vi "CAN Parameters FG.vi"(7 "Action":T1, 8 "error in (no error)":errorcluster, 10 "Diagnostics Basic Configuraiton":T2={"Database File"=path "", "CAN Interface"=enum."CAN0", "Baud Rate"=0, "Diagnostic Protocol"=enum."GMLAN", "Transport Protocol"=enum."ISO TP - Normal Mode", "Transmit ID"=0, "Receive ID"=0, "Transmit Extension"=0, "Receive Extension"=0, "Receive UUDT ID"=0, "Enable Stream"=TRUE, "VW TP Channel ID"=0, "Security"={"Source DLL Path"=path "", "Security Level"=1, "Target DLL Path"=path ""}, "Fill Frame"=TRUE, "Fill Byte"=255, "Termination"=FALSE} {"Fill Byte" format="%.0x"; "VW TP Channel ID" format="%.0x"; "Receive UUDT ID" format="%.0x"; "Receive Extension" format="%.0x"; "Transmit Extension" format="%.0x"; "Receive ID" format="%.0x"; "Transmit ID" format="%.0x"}, 11 "Device Item Ref in":T7 format="%.0x") -> (0 "error out":errorcluster, 2 "Diagnostics Basic Configuraiton":T2={"Database File"=path "", "CAN Interface"=enum."CAN0", "Baud Rate"=0, "Diagnostic Protocol"=enum."GMLAN", "Transport Protocol"=enum."ISO TP - Normal Mode", "Transmit ID"=0, "Receive ID"=0, "Transmit Extension"=0, "Receive Extension"=0, "Receive UUDT ID"=0, "Enable Stream"=TRUE, "VW TP Channel ID"=0, "Security"={"Source DLL Path"=path "", "Security Level"=1, "Target DLL Path"=path ""}, "Fill Frame"=FALSE, "Fill Byte"=255, "Termination"=FALSE} {"Fill Byte" format="%.0x"; "VW TP Channel ID" format="%.0x"; "Receive UUDT ID" format="%.0x"; "Receive Extension" format="%.0x"; "Transmit Extension" format="%.0x"; "Receive ID" format="%.0x"; "Transmit ID" format="%.0x"}, 3 "Device Item Ref out":T7=18446744073709551615 format="%.0x")   [LabVIEW 2015, in "Diagnostics Addon System Explorer.lvlib"]
uses:
  System Explorer/Diagnostics Addon System Explorer.lvlib
  <vilib>/NI Veristand/Custom Device API/Custom Device Item Ref.ctl
  CAN Configuration.ctl
  CAN Interface.ctl
  Diagnostic Protocols.ctl
  Transport Protocols.ctl
  Security.ctl
  FG Action.ctl
  <vilib>/NI Veristand/Custom Device API/Set Item Property (Boolean).vi
  <vilib>/NI Veristand/Custom Device API/Set Item Property (U32).vi
  <vilib>/NI Veristand/Custom Device API/NI VeriStand - Remove Item Property.vi
  <vilib>/NI Veristand/Custom Device API/Set Item Property (Dependent File).vi
  <vilib>/Utility/MD5Checksum.llb/MD5Checksum File.vi
  GUID Lookup.vi
  <vilib>/NI Veristand/Custom Device API/Set Item Property (Path).vi
  <vilib>/NI Veristand/Custom Device API/Get Item Property (Boolean).vi
  <vilib>/NI Veristand/Custom Device API/Get Item Property (U32).vi
  <vilib>/NI Veristand/Custom Device API/Get Item Property (Path).vi
  Diagnostics Addon Shared.lvlib
  <vilib>/NI Veristand/Custom Device API/Custom Device API.lvlib
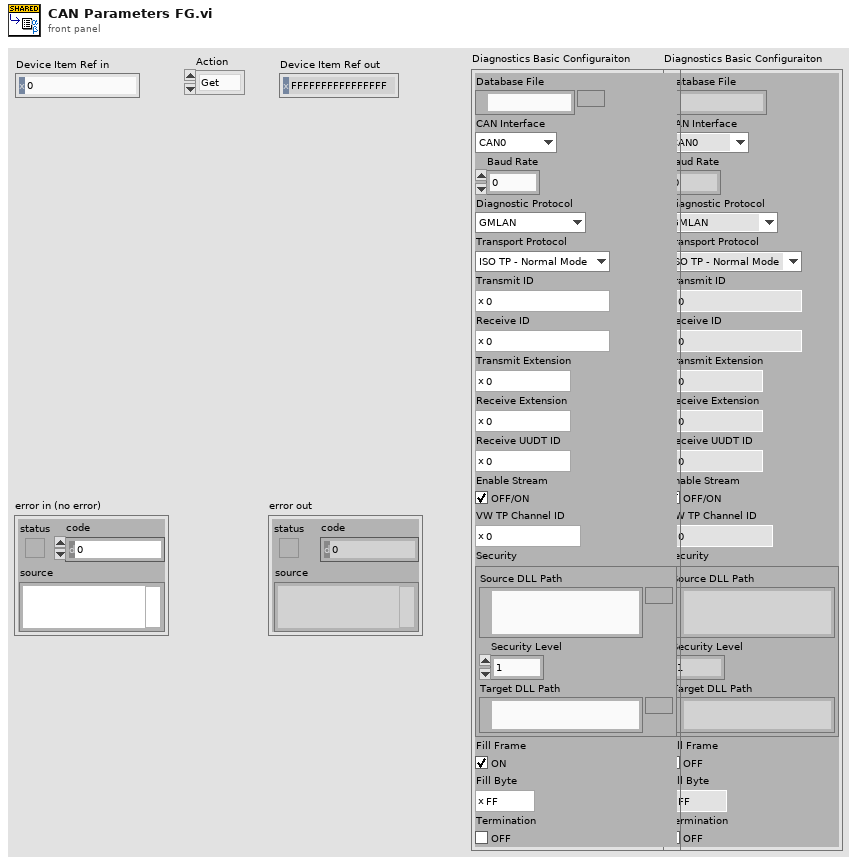
[diagram p1: front panel]
types:
  T1 = typedef "Diagnostics Addon System Explorer.lvlib/FG Action.ctl" = enum16{"Get", "Set"}
  T2 = typedef "Diagnostics Addon Shared.lvlib/CAN Configuration.ctl" = cluster{"Database File":path, "CAN Interface":T3, "Baud Rate":u32, "Diagnostic Protocol":T4, "Transport Protocol":T5, "Transmit ID":u32, "Receive ID":u32, "Transmit Extension":u8, "Receive Extension":u8, "Receive UUDT ID":u32, "Enable Stream":bool, "VW TP Channel ID":u32, "Security":T6, "Fill Frame":bool, "Fill Byte":u8, "Termination":bool}
  T3 = typedef "Diagnostics Addon Shared.lvlib/CAN Interface.ctl" = enum16{"CAN0", "CAN1", "CAN2", "CAN3", "CAN4", "CAN5", "CAN6", "CAN7", "CAN8", "CAN9", "CAN10", "CAN11", "CAN12", "CAN13", "CAN14", "CAN15", "CAN16", "CAN17", "CAN18", "CAN19", "CAN20", "CAN21", "CAN22", "CAN23", "CAN24", "CAN25", "CAN26", "CAN27", "CAN28", "CAN29", "CAN30", "CAN31", "CAN32", "CAN33", "CAN34", "CAN35", "CAN36", "CAN37", "CAN38", "CAN39", "CAN40", "CAN41", "CAN42", "CAN43", "CAN44", "CAN45", "CAN46", "CAN47", "CAN48", "CAN49", "CAN50", "CAN51", "CAN52", "CAN53", "CAN54", "CAN55", "CAN56", "CAN57", "CAN58", "CAN59", "CAN60", "CAN61", "CAN62", "CAN63", "CAN 256 (Virtual)", "CAN 257 (Virtual)"}
  T4 = typedef "Diagnostics Addon Shared.lvlib/Diagnostic Protocols.ctl" = enum16{"GMLAN", "KWP-2000", "UDS"}
  T5 = typedef "Diagnostics Addon Shared.lvlib/Transport Protocols.ctl" = enum16{"ISO TP - Normal Mode", "ISO TP - Mixed Mode", "VW TP 2.0", "Diagnostics on IP"}
  T6 = typedef "Diagnostics Addon Shared.lvlib/Security.ctl" = cluster{"Source DLL Path":path, "Security Level":u8, "Target DLL Path":path}
  T7 = typedef "Custom Device API.lvlib/Custom Device Item Ref.ctl" = u64
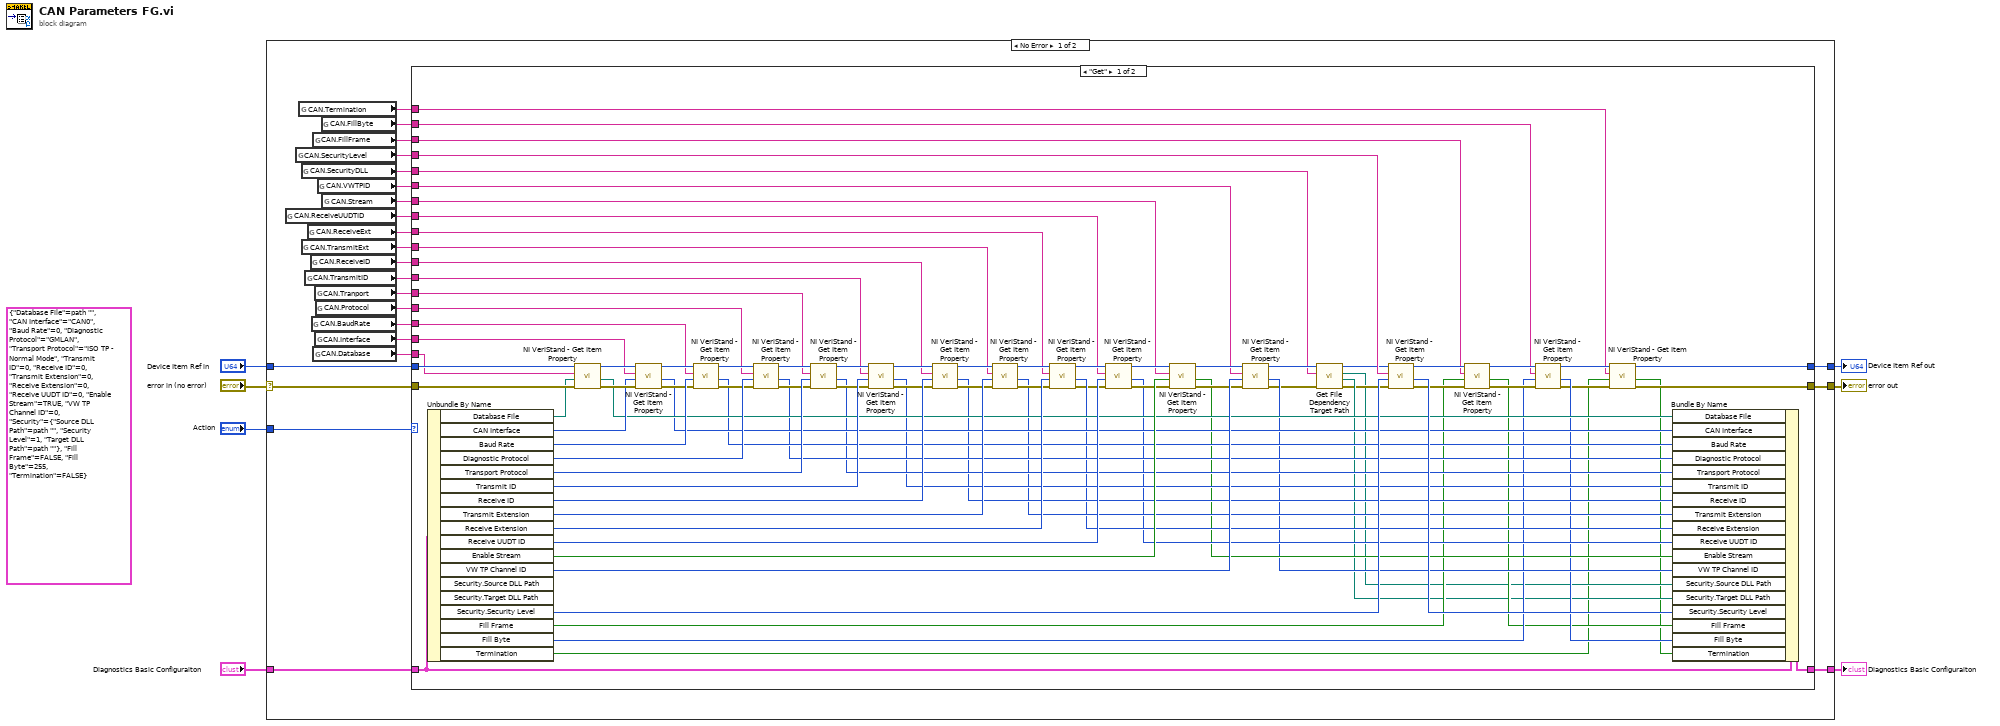
[diagram p0: block diagram]
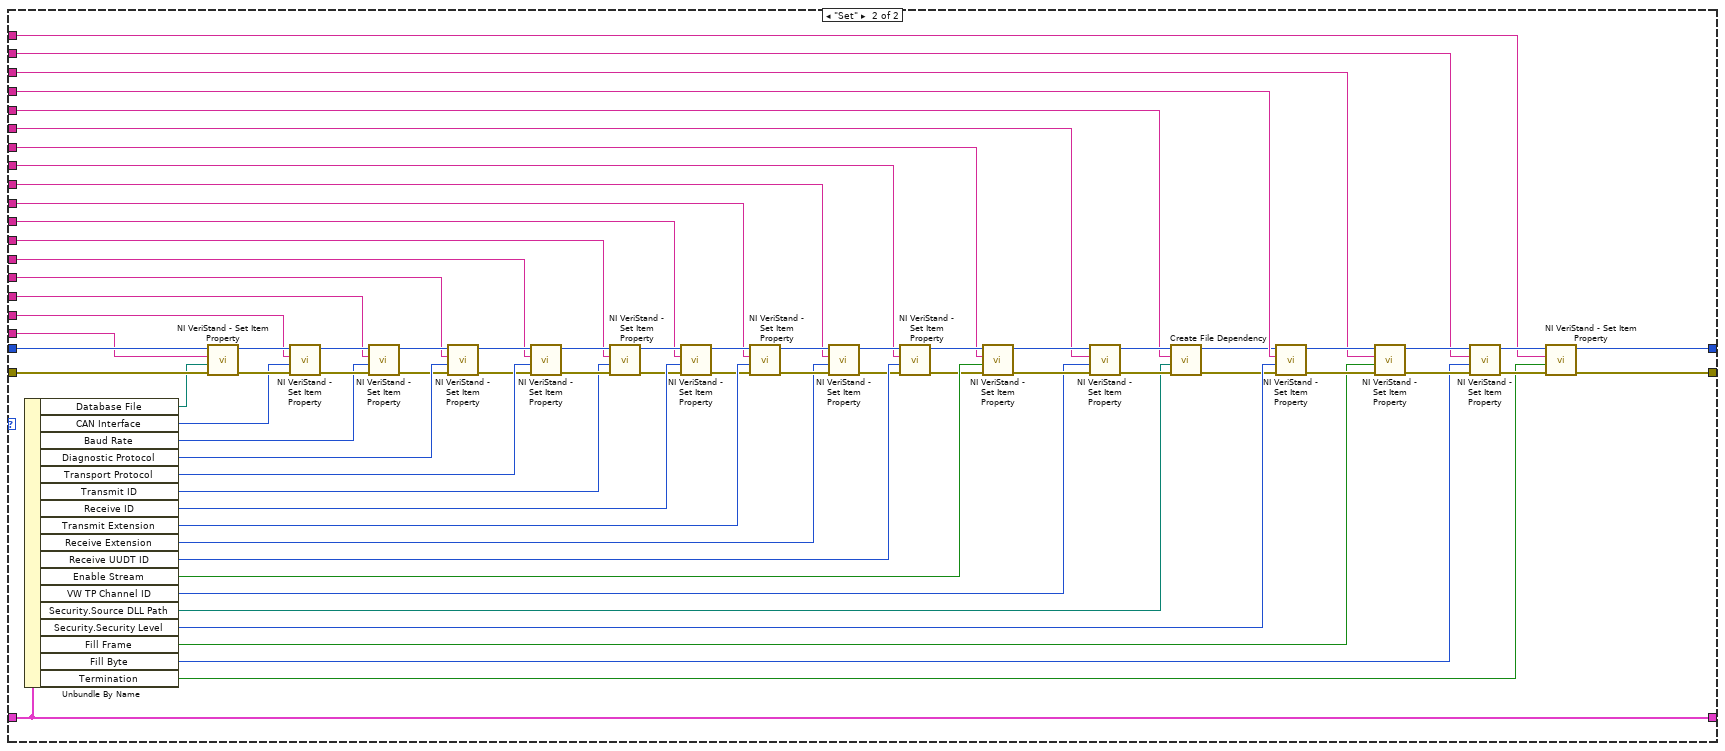
[diagram p2: hidden frame]
diagram:
  (unwired) T2 {"Database File"=path "", "CAN Interface"=enum."CAN0", "Baud Rate"=0, "Diagnostic Protocol"=enum."GMLAN", "Transport Protocol"=enum."ISO TP - Normal Mode", "Transmit ID"=0, "Receive ID"=0, "Transmit Extension"=0, "Receive Extension"=0, "Receive UUDT ID"=0, "Enable Stream"=TRUE, "VW TP Channel ID"=0, "Security"={"Source DLL Path"=path "", "Security Level"=1, "Target DLL Path"=path ""}, "Fill Frame"=FALSE, "Fill Byte"=255, "Termination"=FALSE} ("Diagnostics Basic Configuraiton 2")
  n1 = case shown="No Error" "error in (no error)" {
    selector: "error in (no error)" -> [w31 w192]
    tunnel: "Device Item Ref in" -> [w30 w193]
    tunnel: [w29 w193] -> w4
    tunnel: [w28 w192] -> w5
    tunnel: [w27 _] -> w3
    tunnel: "Diagnostics Basic Configuraiton" -> [w26 _]
    tunnel: "Action" -> [w25 _]
    frame No Error {
      n2 = global read "GUID Lookup.vi" "CAN.ReceiveUUDTID"() -> (w15:string)
      n3 = global read "GUID Lookup.vi" "CAN.SecurityLevel"() -> (w11:string)
      n4 = global read "GUID Lookup.vi" "CAN.Termination"() -> (w8:string)
      n5 = global read "GUID Lookup.vi" "CAN.SecurityDLL"() -> (w12:string)
      n6 = global read "GUID Lookup.vi" "CAN.TransmitExt"() -> (w17:string)
      n7 = global read "GUID Lookup.vi" "CAN.TransmitID"() -> (w19:string)
      n8 = global read "GUID Lookup.vi" "CAN.ReceiveExt"() -> (w16:string)
      n9 = global read "GUID Lookup.vi" "CAN.ReceiveID"() -> (w18:string)
      n10 = global read "GUID Lookup.vi" "CAN.BaudRate"() -> (w22:string)
      n11 = global read "GUID Lookup.vi" "CAN.FillFrame"() -> (w10:string)
      n12 = global read "GUID Lookup.vi" "CAN.Database"() -> (w24:string)
      n13 = global read "GUID Lookup.vi" "CAN.Tranport"() -> (w20:string)
      n14 = global read "GUID Lookup.vi" "CAN.Interface"() -> (w23:string)
      n15 = global read "GUID Lookup.vi" "CAN.Protocol"() -> (w21:string)
      n16 = global read "GUID Lookup.vi" "CAN.VWTPID"() -> (w13:string)
      n17 = global read "GUID Lookup.vi" "CAN.FillByte"() -> (w9:string)
      n18 = global read "GUID Lookup.vi" "CAN.Stream"() -> (w14:string)
      n19 = case shown="\"Get\"" w25 {
        tunnel: w31 -> [w118 w191]
        tunnel: w30 -> [w117 w190]
        tunnel: [w35 w123] -> w29
        tunnel: [w36 w124] -> w28
        tunnel: [w119 w189] -> w27
        tunnel: w26 -> [w120 w189]
        tunnel: w24 -> [w68 w153]
        tunnel: w23 -> [w67 w152]
        tunnel: w22 -> [w66 w151]
        tunnel: w21 -> [w65 w150]
        tunnel: w20 -> [w64 w149]
        tunnel: w19 -> [w63 w148]
        tunnel: w18 -> [w62 w147]
        tunnel: w17 -> [w61 w146]
        tunnel: w16 -> [w60 w145]
        tunnel: w15 -> [w59 w144]
        tunnel: w14 -> [w58 w143]
        tunnel: w13 -> [w57 w142]
        tunnel: w12 -> [w43 w128]
        tunnel: w11 -> [w56 w141]
        tunnel: w10 -> [w47 w130]
        tunnel: w9 -> [w46 w131]
        tunnel: w8 -> [w32 w122]
        frame "Get" {
          n20 = Unbundle By Name(w120) -> ("Database File"=w115:path, "CAN Interface"=w114:T3, "Baud Rate"=w113:u32, "Diagnostic Protocol"=w112:T4, "Transport Protocol"=w111:T5, "Transmit ID"=w110:u32, "Receive ID"=w109:u32, "Transmit Extension"=w108:u8, "Receive Extension"=w107:u8, "Receive UUDT ID"=w106:u32, "Enable Stream"=w105:bool, "VW TP Channel ID"=w104:u32, "Security.Security Level"=w103:u8, "Fill Frame"=w51:bool, "Fill Byte"=w50:u8, "Termination"=w34:bool)  [unwired: 2 out]
          n21 = call-poly <vilib>:"NI VeriStand - Get Item Property.vi"("error in (no error)"=w118, "Default Value"=w115, "Property Name"=w68, "Item Ref in"=w117) -> ("error out"=w116:errorcluster, "Value"=w81:path, "Item Ref out"=w102:T7)  [unwired: 4 in, 1 out]
          n22 = call-poly <vilib>:"NI VeriStand - Get Item Property.vi"("error in (no error)"=w116, "Default Value"=w114, "Property Name"=w67, "Item Ref in"=w102) -> ("error out"=w83:errorcluster, "Value"=w80:u32, "Item Ref out"=w101:T7)  [unwired: 4 in, 1 out]
          n23 = call-poly <vilib>:"NI VeriStand - Get Item Property.vi"("error in (no error)"=w83, "Default Value"=w113, "Property Name"=w66, "Item Ref in"=w101) -> ("error out"=w84:errorcluster, "Value"=w79:u32, "Item Ref out"=w100:T7)  [unwired: 4 in, 1 out]
          n24 = call-poly <vilib>:"NI VeriStand - Get Item Property.vi"("error in (no error)"=w84, "Default Value"=w112, "Property Name"=w65, "Item Ref in"=w100) -> ("error out"=w85:errorcluster, "Value"=w78:u32, "Item Ref out"=w99:T7)  [unwired: 4 in, 1 out]
          n25 = call-poly <vilib>:"NI VeriStand - Get Item Property.vi"("error in (no error)"=w85, "Default Value"=w111, "Property Name"=w64, "Item Ref in"=w99) -> ("error out"=w86:errorcluster, "Value"=w77:u32, "Item Ref out"=w98:T7)  [unwired: 4 in, 1 out]
          n26 = call-poly <vilib>:"NI VeriStand - Get Item Property.vi"("error in (no error)"=w86, "Default Value"=w110, "Property Name"=w63, "Item Ref in"=w98) -> ("error out"=w87:errorcluster, "Value"=w76:u32, "Item Ref out"=w97:T7)  [unwired: 4 in, 1 out]
          n27 = call-poly <vilib>:"NI VeriStand - Get Item Property.vi"("error in (no error)"=w87, "Default Value"=w109, "Property Name"=w62, "Item Ref in"=w97) -> ("error out"=w88:errorcluster, "Value"=w75:u32, "Item Ref out"=w96:T7)  [unwired: 4 in, 1 out]
          n28 = call-poly <vilib>:"NI VeriStand - Get Item Property.vi"("error in (no error)"=w88, "Default Value"=w108, "Property Name"=w61, "Item Ref in"=w96) -> ("error out"=w89:errorcluster, "Value"=w74:u32, "Item Ref out"=w95:T7)  [unwired: 4 in, 1 out]
          n29 = call-poly <vilib>:"NI VeriStand - Get Item Property.vi"("error in (no error)"=w89, "Default Value"=w107, "Property Name"=w60, "Item Ref in"=w95) -> ("error out"=w72:errorcluster, "Value"=w73:u32, "Item Ref out"=w94:T7)  [unwired: 4 in, 1 out]
          n30 = call-poly <vilib>:"NI VeriStand - Get Item Property.vi"("error in (no error)"=w72, "Default Value"=w106, "Property Name"=w59, "Item Ref in"=w94) -> ("error out"=w90:errorcluster, "Value"=w71:u32, "Item Ref out"=w93:T7)  [unwired: 4 in, 1 out]
          n31 = call-poly <vilib>:"NI VeriStand - Get Item Property.vi"("error in (no error)"=w90, "Default Value"=w105, "Property Name"=w58, "Item Ref in"=w93) -> ("error out"=w91:errorcluster, "Value"=w70:bool, "Item Ref out"=w92:T7)  [unwired: 4 in, 1 out]
          n32 = call-poly <vilib>:"NI VeriStand - Get Item Property.vi"("error in (no error)"=w91, "Default Value"=w104, "Property Name"=w57, "Item Ref in"=w92) -> ("error out"=w44:errorcluster, "Value"=w69:u32, "Item Ref out"=w45:T7)  [unwired: 4 in, 1 out]
          n33 = call "Get File Dependency Target Path.vi"("error in (no error)"=w44, "Bitfile 986x"=w43, "Item Ref in"=w45) -> ("error out"=w41:errorcluster, "Target Path"=w42:path, "Source Path"=w39:path, "Item Ref out"=w40:T7)  [unwired: 5 in]
          n34 = call-poly <vilib>:"NI VeriStand - Get Item Property.vi"("error in (no error)"=w41, "Default Value"=w103, "Property Name"=w56, "Item Ref in"=w40) -> ("error out"=w53:errorcluster, "Value"=w82:u32, "Item Ref out"=w52:T7)  [unwired: 4 in, 1 out]
          n35 = call-poly <vilib>:"NI VeriStand - Get Item Property.vi"("error in (no error)"=w53, "Default Value"=w51, "Property Name"=w47, "Item Ref in"=w52) -> ("error out"=w55:errorcluster, "Value"=w48:bool, "Item Ref out"=w54:T7)  [unwired: 4 in, 1 out]
          n36 = call-poly <vilib>:"NI VeriStand - Get Item Property.vi"("error in (no error)"=w55, "Default Value"=w50, "Property Name"=w46, "Item Ref in"=w54) -> ("error out"=w37:errorcluster, "Value"=w49:u32, "Item Ref out"=w38:T7)  [unwired: 4 in, 1 out]
          n37 = call-poly <vilib>:"NI VeriStand - Get Item Property.vi"("error in (no error)"=w37, "Default Value"=w34, "Property Name"=w32, "Item Ref in"=w38) -> ("error out"=w36:errorcluster, "Value"=w33:bool, "Item Ref out"=w35:T7)  [unwired: 4 in, 1 out]
          n38 = Bundle By Name(cluster=w120, "Database File"=w81, "CAN Interface"=w80, "Baud Rate"=w79, "Diagnostic Protocol"=w78, "Transport Protocol"=w77, "Transmit ID"=w76, "Receive ID"=w75, "Transmit Extension"=w74, "Receive Extension"=w73, "Receive UUDT ID"=w71, "Enable Stream"=w70, "VW TP Channel ID"=w69, "Security.Source DLL Path"=w39, "Security.Target DLL Path"=w42, "Security.Security Level"=w82, "Fill Frame"=w48, "Fill Byte"=w49, "Termination"=w33) -> (w119:T2)
        }
        frame "Set" {
          n39 = Unbundle By Name(w189) -> ("Database File"=w188:path, "CAN Interface"=w185:T3, "Baud Rate"=w182:u32, "Diagnostic Protocol"=w175:T4, "Transport Protocol"=w174:T5, "Transmit ID"=w173:u32, "Receive ID"=w172:u32, "Transmit Extension"=w171:u8, "Receive Extension"=w170:u8, "Receive UUDT ID"=w169:u32, "Enable Stream"=w168:bool, "VW TP Channel ID"=w167:u32, "Security.Source DLL Path"=w127:path, "Security.Security Level"=w166:u8, "Fill Frame"=w133:bool, "Fill Byte"=w132:u8, "Termination"=w121:bool)
          n40 = call-poly <vilib>:"NI VeriStand - Set Item Property.vi"("error in (no error)"=w191, "Value"=w188, "Property Name"=w153, "Item Ref in"=w190) -> ("error out"=w186:errorcluster, "Item Ref out"=w187:T7)  [unwired: 5 in, 1 out]
          n41 = call-poly <vilib>:"NI VeriStand - Set Item Property.vi"("error in (no error)"=w186, "Value"=w185, "Property Name"=w152, "Item Ref in"=w187) -> ("error out"=w183:errorcluster, "Item Ref out"=w184:T7)  [unwired: 5 in, 1 out]
          n42 = call-poly <vilib>:"NI VeriStand - Set Item Property.vi"("error in (no error)"=w183, "Value"=w182, "Property Name"=w151, "Item Ref in"=w184) -> ("error out"=w154:errorcluster, "Item Ref out"=w165:T7)  [unwired: 5 in, 1 out]
          n43 = call-poly <vilib>:"NI VeriStand - Set Item Property.vi"("error in (no error)"=w154, "Value"=w175, "Property Name"=w150, "Item Ref in"=w165) -> ("error out"=w155:errorcluster, "Item Ref out"=w164:T7)  [unwired: 5 in, 1 out]
          n44 = call-poly <vilib>:"NI VeriStand - Set Item Property.vi"("error in (no error)"=w155, "Value"=w174, "Property Name"=w149, "Item Ref in"=w164) -> ("error out"=w181:errorcluster, "Item Ref out"=w180:T7)  [unwired: 5 in, 1 out]
          n45 = call-poly <vilib>:"NI VeriStand - Set Item Property.vi"("error in (no error)"=w181, "Value"=w173, "Property Name"=w148, "Item Ref in"=w180) -> ("error out"=w156:errorcluster, "Item Ref out"=w163:T7)  [unwired: 5 in, 1 out]
          n46 = call-poly <vilib>:"NI VeriStand - Set Item Property.vi"("error in (no error)"=w156, "Value"=w172, "Property Name"=w147, "Item Ref in"=w163) -> ("error out"=w157:errorcluster, "Item Ref out"=w162:T7)  [unwired: 5 in, 1 out]
          n47 = call-poly <vilib>:"NI VeriStand - Set Item Property.vi"("error in (no error)"=w157, "Value"=w171, "Property Name"=w146, "Item Ref in"=w162) -> ("error out"=w177:errorcluster, "Item Ref out"=w176:T7)  [unwired: 5 in, 1 out]
          n48 = call-poly <vilib>:"NI VeriStand - Set Item Property.vi"("error in (no error)"=w177, "Value"=w170, "Property Name"=w145, "Item Ref in"=w176) -> ("error out"=w158:errorcluster, "Item Ref out"=w161:T7)  [unwired: 5 in, 1 out]
          n49 = call-poly <vilib>:"NI VeriStand - Set Item Property.vi"("error in (no error)"=w158, "Value"=w169, "Property Name"=w144, "Item Ref in"=w161) -> ("error out"=w159:errorcluster, "Item Ref out"=w160:T7)  [unwired: 5 in, 1 out]
          n50 = call-poly <vilib>:"NI VeriStand - Set Item Property.vi"("error in (no error)"=w159, "Value"=w168, "Property Name"=w143, "Item Ref in"=w160) -> ("error out"=w178:errorcluster, "Item Ref out"=w179:T7)  [unwired: 5 in, 1 out]
          n51 = call-poly <vilib>:"NI VeriStand - Set Item Property.vi"("error in (no error)"=w178, "Value"=w167, "Property Name"=w142, "Item Ref in"=w179) -> ("error out"=w136:errorcluster, "Item Ref out"=w129:T7)  [unwired: 5 in, 1 out]
          n52 = call "Create File Dependency.vi"("error in (no error)"=w136, "DLL Path"=w127, "DLL Property Name"=w128, "Item Ref in"=w129) -> ("error out"=w135:errorcluster, "Item Ref out"=w134:T7)  [unwired: 6 in]
          n53 = call-poly <vilib>:"NI VeriStand - Set Item Property.vi"("error in (no error)"=w135, "Value"=w166, "Property Name"=w141, "Item Ref in"=w134) -> ("error out"=w139:errorcluster, "Item Ref out"=w137:T7)  [unwired: 5 in, 1 out]
          n54 = call-poly <vilib>:"NI VeriStand - Set Item Property.vi"("error in (no error)"=w139, "Value"=w133, "Property Name"=w130, "Item Ref in"=w137) -> ("error out"=w140:errorcluster, "Item Ref out"=w138:T7)  [unwired: 5 in, 1 out]
          n55 = call-poly <vilib>:"NI VeriStand - Set Item Property.vi"("error in (no error)"=w140, "Value"=w132, "Property Name"=w131, "Item Ref in"=w138) -> ("error out"=w126:errorcluster, "Item Ref out"=w125:T7)  [unwired: 5 in, 1 out]
          n56 = call-poly <vilib>:"NI VeriStand - Set Item Property.vi"("error in (no error)"=w126, "Value"=w121, "Property Name"=w122, "Item Ref in"=w125) -> ("error out"=w124:errorcluster, "Item Ref out"=w123:T7)  [unwired: 5 in, 1 out]
        }
      }
    }
    frame Error {
    }
  }
  "error out" <- w5
  "Device Item Ref out" <- w4
  "Diagnostics Basic Configuraiton" <- w3
